vi "disable_motion.vi"(8 "error in (no error)":errorcluster caption="错误输入（无错误）", 11 "OneMotion 输入":refnum<class "OneMotion.lvclass">) -> (0 "error out":errorcluster caption="错误输出", 3 "OneMotion 输出":refnum<class "OneMotion.lvclass">)   [LabVIEW 2016, in "MotionControl_UFO_3DOF.lvlib" / "OneMotion.lvclass"]
uses:
  <userlib>/MotionControl_UFO_3DOF/OneMotion/OneMotion.lvclass
  <userlib>/MotionControl_UFO_3DOF/OneMotion/OneMotion.lvclass/OneMotion.ctl
  <userlib>/MotionControl_UFO_3DOF/StepMotor/StepMotor.lvclass
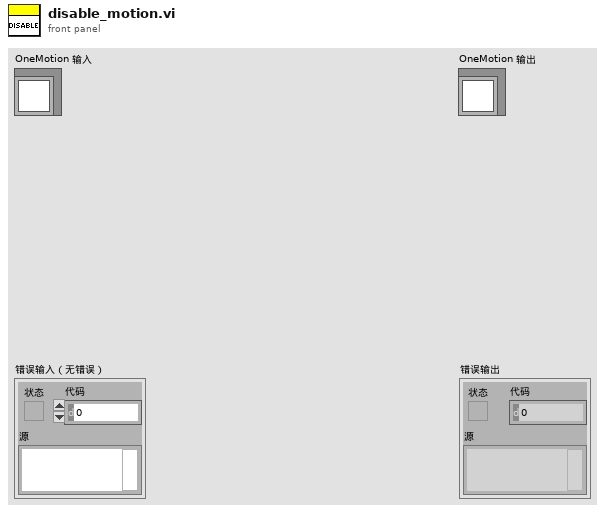
[diagram p1: front panel]
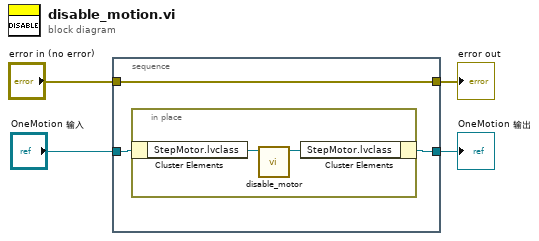
[diagram p0: block diagram]
diagram:
  n1 = stacked-sequence {
    tunnel: [w7] -> w4
    tunnel: [w5] -> w2
    tunnel: "OneMotion 输入" -> [w6]
    tunnel: "error in (no error)" -> [w7]
    frame #0 {
      n2 = in-place {
        n3 = in-place-cluster #1(w6) -> ("StepMotor.lvclass"=w9:refnum<class "StepMotor.lvclass">)
        n4 = call-dynamic "disable_motor.vi"("StepMotor输入"=w9) -> ("StepMotor输出"=w8:refnum<class "StepMotor.lvclass">)  [unwired: 9 in, 1 out]
        n5 = in-place-cluster #1("StepMotor.lvclass"=w8) -> (w5:refnum<class "OneMotion.lvclass">)
      }
    }
  }
  "error out" <- w4
  "OneMotion 输出" <- w2
